vi "Update State.vi"(8 "H":T1, 9 "K":T1, 10 "Observations":T1, 11 "Old State":T1) -> (3 "Updated State":T1)   [LabVIEW 2020]
uses:
  <vilib>/Analysis/Matrix/Datatypes/RealMatrix.ctl
  <vilib>/Analysis/baseanly.llb/Real A x B.vi
  <vilib>/Analysis/Matrix/Numeric/Subtract/Subtract - RM,RM.vi
  <vilib>/Analysis/Matrix/Numeric/Add/Add - RM,RM.vi
  <vilib>/Analysis/NI_AALBase.lvlib
  <vilib>/Analysis/Matrix/NI_Matrix.lvlib
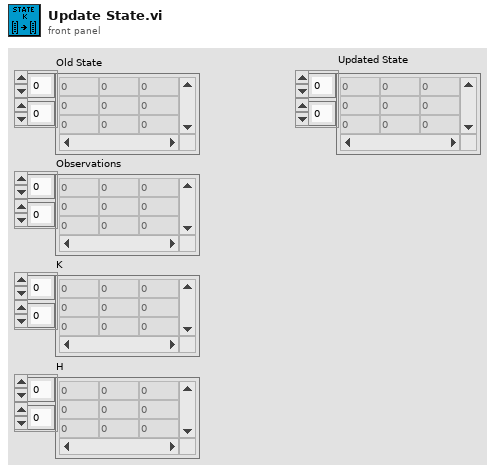
[diagram p1: front panel]
types:
  T1 = typedef "NI_Matrix.lvlib/RealMatrix.ctl" = dbl[][]
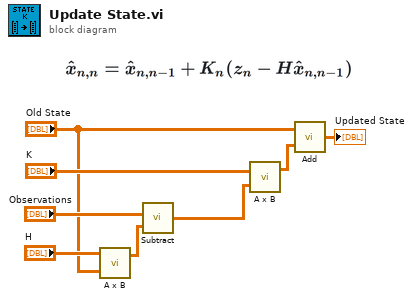
[diagram p0: block diagram]
diagram:
  n1 = call-poly <vilib>:"A x B.vi"("B"="Old State", "A"="H") -> ("A x B"=w5:T1)  [unwired: 1 out]
  n2 = call-poly <vilib>:"Subtract.vi"("Real Matrix B"=w5, "Real Matrix A"="Observations") -> ("A - B"=w4:T1)
  n3 = call-poly <vilib>:"A x B.vi"("B"=w4, "A"="K") -> ("A x B"=w3:T1)  [unwired: 1 out]
  n4 = call-poly <vilib>:"Add.vi"("Real Matrix B"=w3, "Real Matrix A"="Old State") -> ("A + B"=→"Updated State":T1)
